vi "dvp Vi Get Mono State.vi"(10 "pMonoState":i32, 11 "handle":u32) -> (2 "pMonoState out":i32, 3 "function return":u32(ring))   [LabVIEW 2018, in "LabViewDVPCamera.lvlib"]
doc: "LabviewDvp2Api dvpStatus dvpViGetMonoState(dvpHandle handle, BOOL *pMonoState);"
uses:
  LabViewDVPCamera.lvlib
  LabViewDVPCamera/LabViewDVPCamera.dll
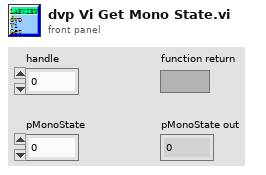
[diagram p1: front panel]
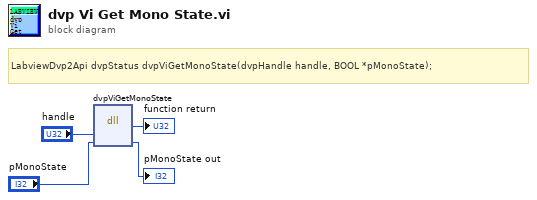
[diagram p0: block diagram]
diagram:
  # "LabviewDvp2Api dvpStatus dvpViGetMonoState(dvpHandle handle, BOOL *pMonoState);"
  n1 = dll-call lib="C:/Program Files (x86)/DVP2 Labview cn 64/Sample/LabViewDVPCamera/LabViewDVPCamera.*" fn="dvpViGetMonoState"("handle"="handle", "pMonoState"="pMonoState") -> (→"function return":u32, "pMonoState"=→"pMonoState out":i32)  [unwired: 4 in, 2 out]
